vi "Average.vi"(9 "Transparency Factor":dbl=0.5, 10 "x":u8, 11 "y":u8) -> (3 "z":u8)   [LabVIEW 2012, in "Picture Box Tools.lvlib"]
uses:
  Picture Box Tools.lvlib
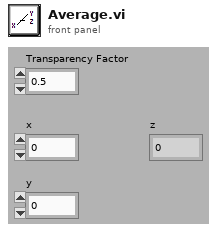
[diagram p1: front panel]
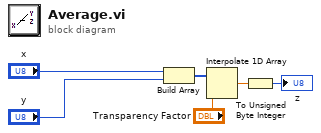
[diagram p0: block diagram]
diagram:
  n1 = Build Array("x", "y") -> (w1:u8[])
  n2 = Interpolate 1D Array(1:"Transparency Factor", 2:w1) -> (0:w3:dbl)
  n3 = To Unsigned Byte Integer(number=w3) -> (unsigned 8bit integer=→"z":u8)
